vi "Test RT Interpreter API-RT.vi"() -> ()   [LabVIEW 2021]
doc: "RT Interpreter API Tester for Real-Time."
uses:
  Host/Host Interpreter/Host Initialization--cluster.ctl
  Libraries/UDP Comms/UDP Message--cluster.ctl
  <vilib>/Utility/error.llb/DialogType.ctl
  RT Interpreter.lvlib
  Libraries/Common RT/Common RT.lvlib
  Libraries/UDP Comms/UDP Comms.lvlib
panel:
  in  "UDP Message":T1
  in  "Send Message to Host":bool
  in  "Host Initialization--cluster":T2
  out "List of IP:Port:Master/Slave":string[](array[string])
  in  "Exit":bool
  in  "Refresh Modules":bool
  in  "Stop Module Instance":bool
  in  "Run New Module Instance":bool
  out "error out":errorcluster
  out "last error":errorcluster
  out "Active Modules":string[](array[string])
  in  "Select Module":i32(ring)=-1 caption="Select Module\nTo send Request to" items=["All"=-1, "1"=1]
  out "Status":string
  # "This VI tests the API for the Module."
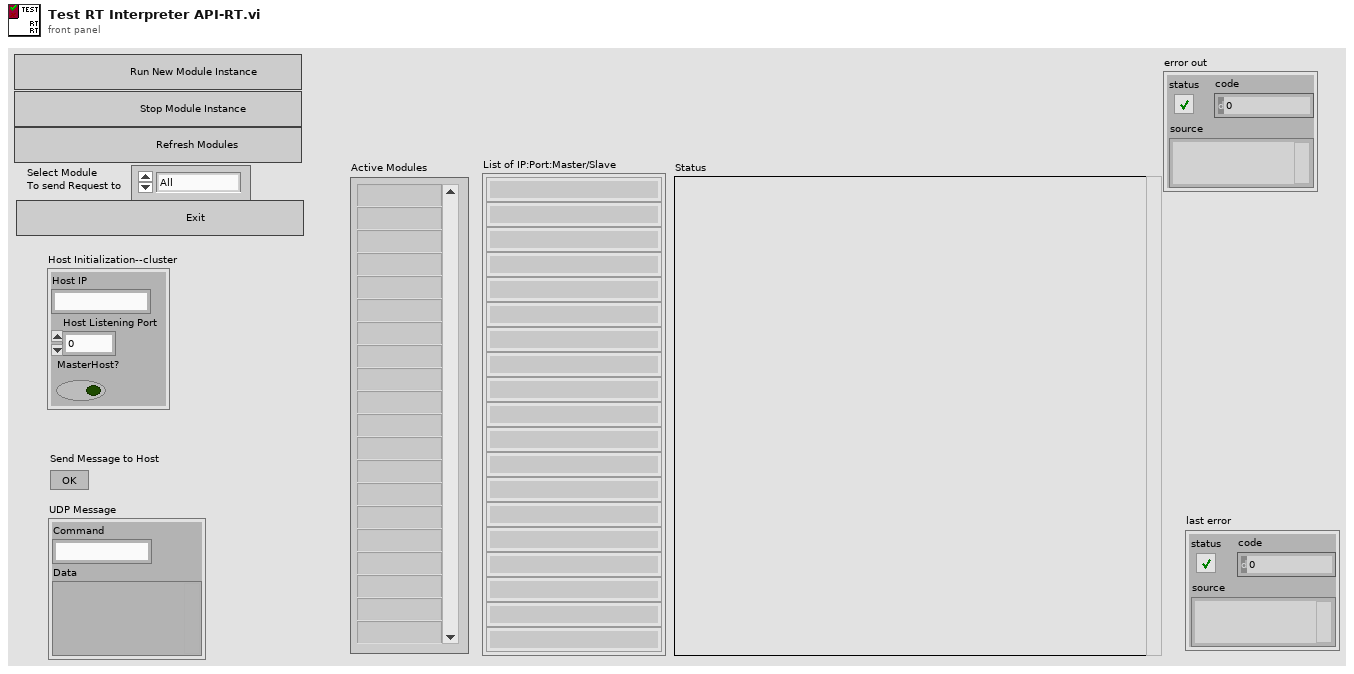
[diagram p1: front panel]
types:
  T1 = typedef "UDP Comms.lvlib/UDP Message--cluster.ctl" = cluster{"Command":string, "Data":variant}
  T2 = typedef "UDP Comms.lvlib/Host Initialization--cluster.ctl" = cluster{"Host IP":string, "Host Listening Port":u16, "MasterHost?":bool}
  T3 = typedef "RT Interpreter.lvlib/Broadcast Events--cluster.ctl" = cluster{"Module Did Init":refnum<user-event>, "Status Updated":refnum<user-event>, "Error Reported":refnum<user-event>, "Module Did Stop":refnum<user-event>, "Update Module Execution Status":refnum<user-event>}
  T4 = typedef "DialogType.ctl" = u16
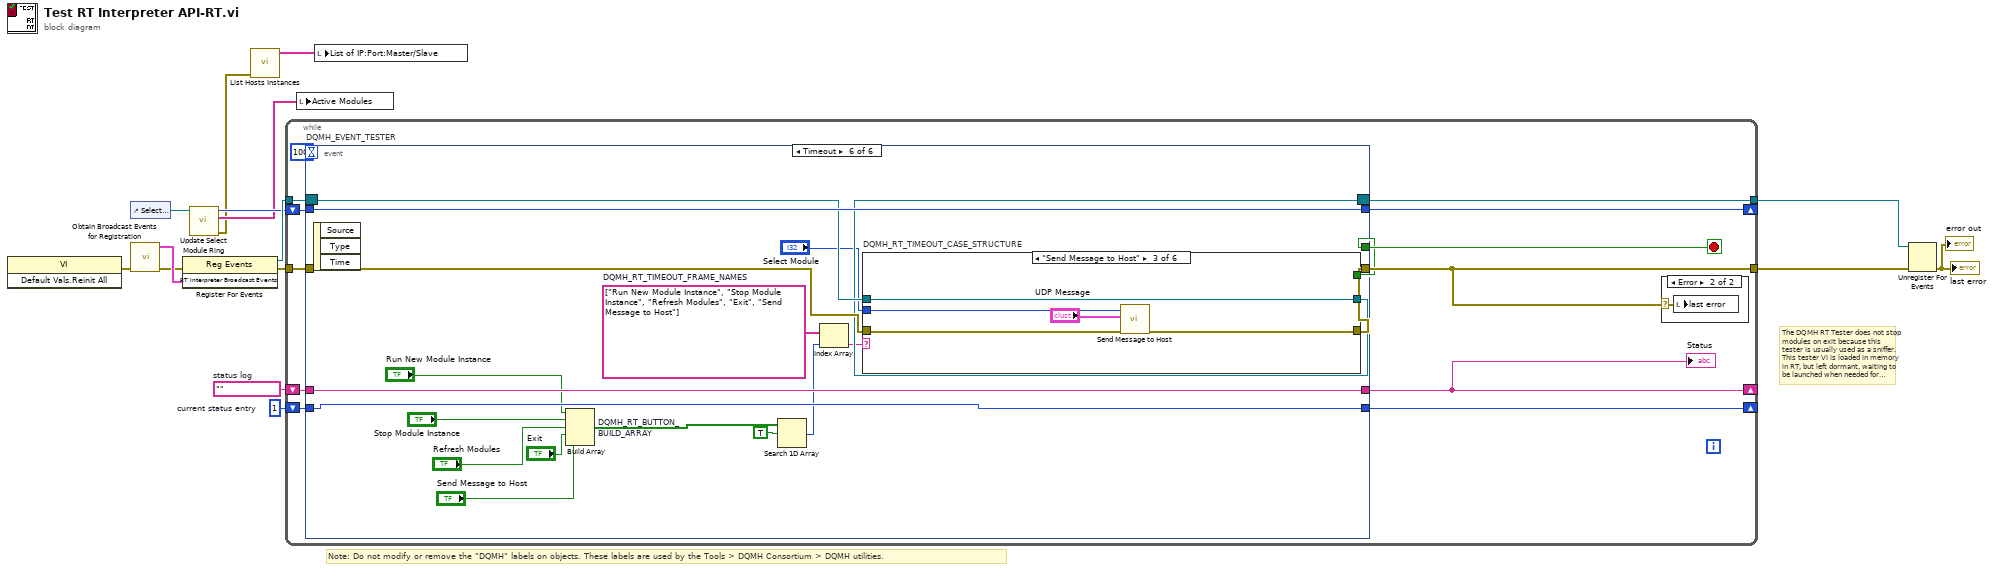
[diagram p0: block diagram]
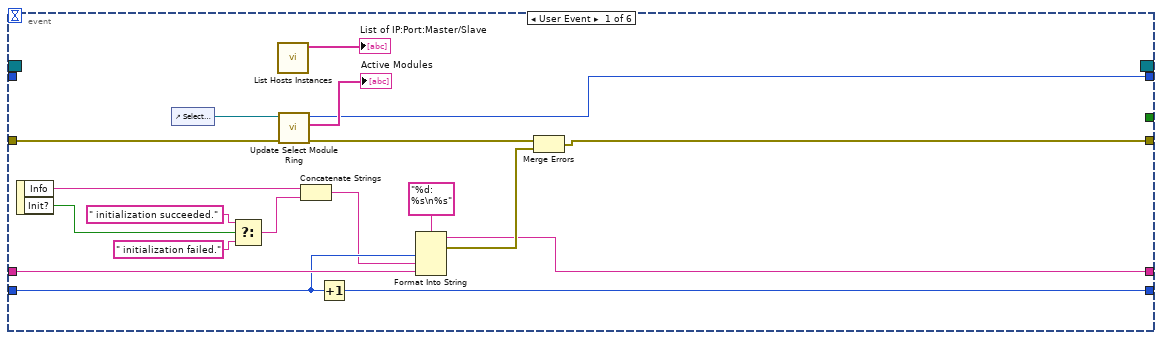
[diagram p3: hidden frame]
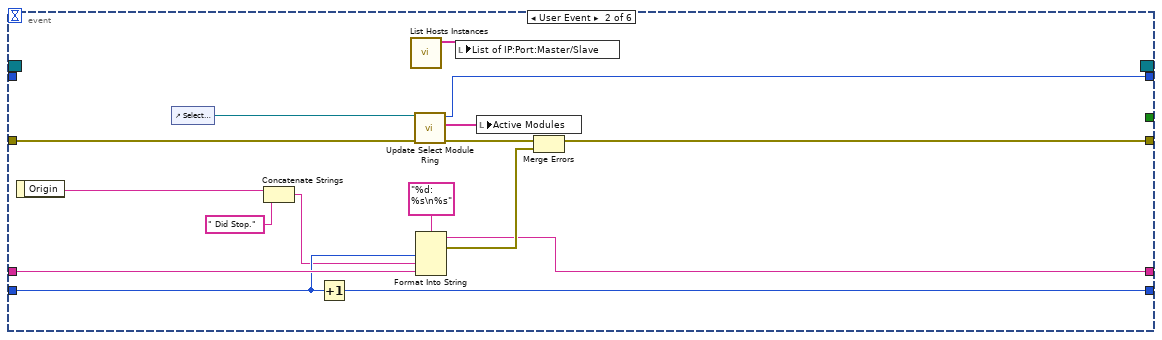
[diagram p4: hidden frame]
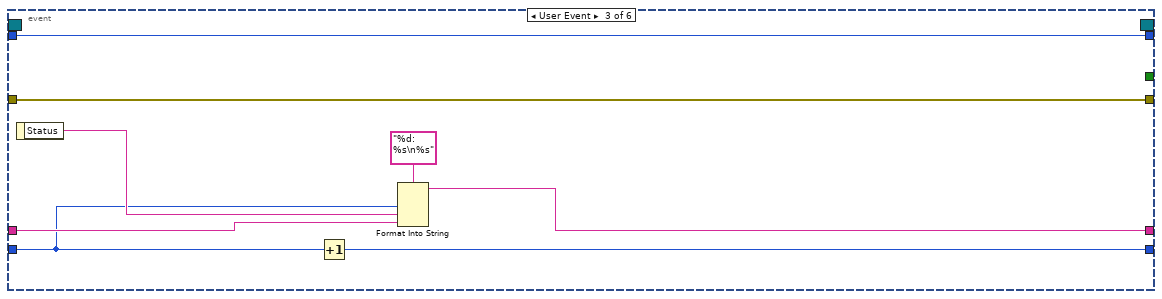
[diagram p5: hidden frame]
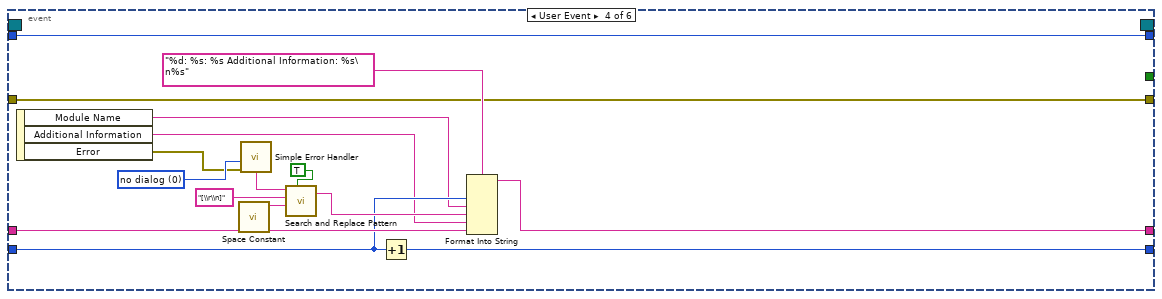
[diagram p6: hidden frame]
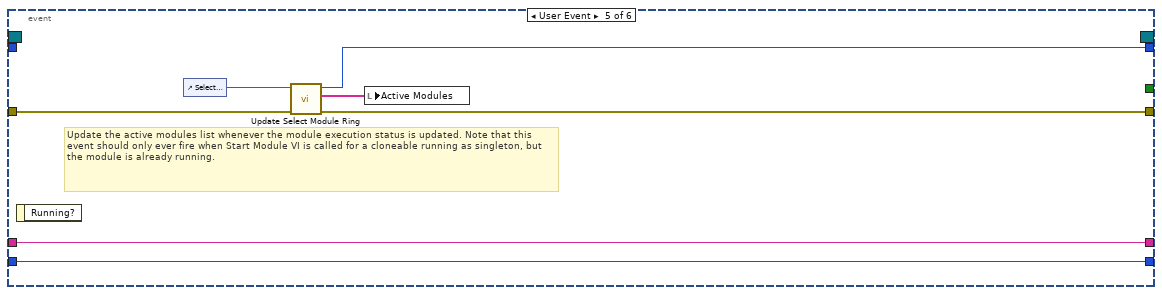
[diagram p7: hidden frame]
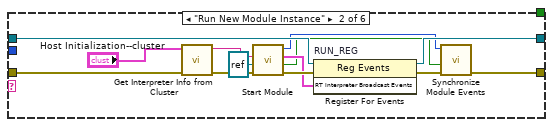
[diagram p9: hidden frame]
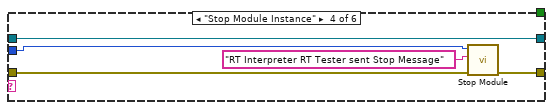
[diagram p10: hidden frame]
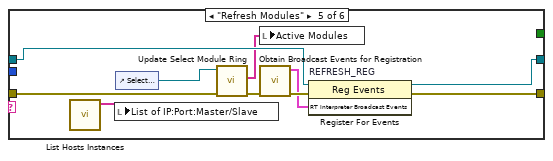
[diagram p11: hidden frame]
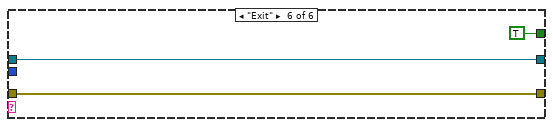
[diagram p12: hidden frame]
diagram:
  w13 = 1  # current status entry
  w14 = ""  # status log
  # "The DQMH RT Tester does not stop modules on exit because this tester is usually used as a sniffer. This tester VI is loaded in memory in RT, but left dormant, waiting to be launched when needed for troubleshooting."
  # "Note: Do not modify or remove the \"DQMH\" labels on objects. These labels are used by the Tools > DQMH Consortium > DQMH utilities."
  n1 = invoke class="VI" method="Default Vals.Reinit All"() -> (error out=w9:errorcluster)  [unwired: 3 in, 2 out]
  n2 = control-ref of="Select Module"() -> (w5:refnum<vi>)
  n3 = call "Obtain Broadcast Events for Registration.vi"("error in"=w9) -> ("error out"=w8:errorcluster, "RT Interpreter Broadcast Events"=w12:T3)  [unwired: 8 in, 1 out]
  n4 = register-events(error in=w8, w12) -> (reference out=w15:refnum<event-registration>, error out=w11:errorcluster)  [unwired: 1 in]
  n5 = call "Update Select Module Ring.vi"("Select Module Ring Ref"=w5) -> ("error out"=w1:errorcluster, "Active Modules (Array)"=w3:string[], "New Module Ring Value"=w4:i32)  [unwired: 8 in]
  n6 = call "List Hosts Instances.vi"("error in"=w1) -> ("List of IP:Port:Master/Slave"=w2:string[])  [unwired: 9 in, 1 out]
  n7 = while {
    tunnel: w15 -> [w27]
    tunnel: [w18] -> w7
    tunnel: w11 -> [w26]
    shift-right: [w22] -> _
    shift-left: w14 -> [w24]
    shift-right: [w23] -> _
    shift-left: w13 -> [w25]
    shift-right: [w20] -> _
    shift-left: w4 -> [w21]
    tunnel: [w19] -> w10
    stop <- w17 stop-if-true
    n8 = event "DQMH_EVENT_TESTER" shown="[5] Timeout" {
      selector: w27 -> [_ _ _ _ _ w108]
      dyn-events: [_ _ _ _ _ w107] -> w19
      timeout: 100 -> [_ _ _ _ _ _]
      tunnel: [_ _ _ _ _ w101] -> w17
      tunnel: [w37 w55 w71 w75 w90 w109] -> w18
      tunnel: w26 -> [w39 w57 w71 w75 w91 w113]
      tunnel: w25 -> [w44 w60 w64 w78 w93 w111]
      tunnel: w24 -> [w45 w61 w67 w79 w94 w112]
      tunnel: [w42 w58 w68 w77 w94 w112] -> w22
      tunnel: [w43 w59 w70 w76 w93 w111] -> w23
      tunnel: w21 -> [_ _ w65 w87 _ w110]
      tunnel: [w34 w52 w65 w87 w89 w110] -> w20
      event User Event {
        n9 = event-data() -> ("Info"=w41:string, "Init?"=w31:bool)  [unwired: 1 in]
        n10 = control-ref of="Select Module"() -> (w36:refnum<vi>)
        n11 = Select(t=" initialization succeeded.", s=w31, f=" initialization failed.") -> (s? t:f=w30:string)
        n12 = call "List Hosts Instances.vi"() -> ("List of IP:Port:Master/Slave"=→"List of IP:Port:Master/Slave":string[])  [unwired: 10 in, 1 out]
        n13 = call "Update Select Module Ring.vi"("error in"=w39, "Select Module Ring Ref"=w36) -> ("error out"=w38:errorcluster, "Active Modules (Array)"=→"Active Modules":string[], "New Module Ring Value"=w34:i32)  [unwired: 7 in]
        n14 = Concatenate Strings(w41, w30) -> (w40:string)
        n15 = Increment(x=w44) -> (x+1=w43:i32)
        n16 = Format Into String(format string="%d: %s\n%s", w44, w40, w45) -> (resulting string=w42:string, error out=w47:errorcluster)  [unwired: 2 in]
        n17 = Merge Errors(w38, w47) -> (w37:errorcluster)
      }
      event User Event {
        n18 = event-data() -> ("Origin"=w50:string)  [unwired: 1 in]
        n19 = control-ref of="Select Module"() -> (w54:refnum<vi>)
        n20 = Concatenate Strings(w50, " Did Stop.") -> (w49:string)
        n21 = Increment(x=w60) -> (x+1=w59:i32)
        n22 = call "List Hosts Instances.vi"() -> ("List of IP:Port:Master/Slave"=w48:string[])  [unwired: 10 in, 1 out]
        n23 = call "Update Select Module Ring.vi"("error in"=w57, "Select Module Ring Ref"=w54) -> ("error out"=w56:errorcluster, "Active Modules (Array)"=w53:string[], "New Module Ring Value"=w52:i32)  [unwired: 7 in]
        n24 = Format Into String(format string="%d: %s\n%s", w60, w49, w61) -> (resulting string=w58:string, error out=w63:errorcluster)  [unwired: 2 in]
        n25 = local write "List of IP:Port:Master/Slave"(w48) -> ()
        n26 = local write "Active Modules"(w53) -> ()
        n27 = Merge Errors(w56, w63) -> (w55:errorcluster)
      }
      event User Event {
        n28 = event-data() -> ("Status"=w66:string)  [unwired: 1 in]
        n29 = Increment(x=w64) -> (x+1=w70:i32)
        n30 = Format Into String(format string="%d: %s\n%s", w64, w66, w67) -> (resulting string=w68:string)  [unwired: 2 in, 1 out]
      }
      event User Event {
        w80 = T4 0 items=["no dialog", "OK message", "continue or stop message", "OK message + warnings", "continue/stop + warnings"] ("type of dialog (OK msg:1)")
        n31 = event-data() -> ("Module Name"=w74:string, "Additional Information"=w73:string, "Error"=w72:errorcluster)  [unwired: 1 in]
        n32 = call <vilib>:"Space Constant.vi"() -> ("String"=w84:string)
        n33 = call <vilib>:"Simple Error Handler.vi"("type of dialog (OK msg:1)"=w80, "error in (no error)"=w72) -> ("message"=w81:string)  [unwired: 3 in, 4 out]
        n34 = call <vilib>:"Search and Replace Pattern.vi"("string"=w81, "regular expression (\"\")"="[\\r\\n]" ("regular expression (\"\")"), "replace string (\"\")"=w84, "replace all? (F)"=TRUE ("replace all CR/LF with spaces")) -> ("result string"=w82:string)  [unwired: 1 in, 1 out]
        n35 = Increment(x=w78) -> (x+1=w76:i32)
        n36 = Format Into String(format string="%d: %s: %s Additional Information: %s\n%s", w78, w74, w82, w73, w79) -> (resulting string=w77:string)  [unwired: 2 in, 1 out]
      }
      event User Event {
        # "Update the active modules list whenever the module execution status is updated. Note that this event should only ever fire when Start Module VI is called for a cloneable running as singleton, but the module is already running."
        n37 = event-data() -> ()  [unwired: 1 in, 1 out]
        n38 = control-ref of="Select Module"() -> (w92:refnum<vi>)
        n39 = call "Update Select Module Ring.vi"("error in"=w91, "Select Module Ring Ref"=w92) -> ("error out"=w90:errorcluster, "Active Modules (Array)"=w88:string[], "New Module Ring Value"=w89:i32)  [unwired: 7 in]
        n40 = local write "Active Modules"(w88) -> ()
      }
      event Timeout {
        w99 = string[] ["Run New Module Instance", "Stop Module Instance", "Refresh Modules", "Exit", "Send Message to Host"]  # DQMH_RT_TIMEOUT_FRAME_NAMES
        n41 = event-data() -> ()  [unwired: 1 in, 3 out]
        n42 = Build Array "DQMH_RT_BUTTON_BUILD_ARRAY"("Run New Module Instance", "Stop Module Instance", "Refresh Modules", "Exit", "Send Message to Host") -> (w96:bool[])
        n43 = Search 1D Array(1D array=w96, element=TRUE) -> (index of element=w98:i32)  [unwired: 1 in]
        n44 = Index Array(array=w99, index=w98) -> (element=w100:string)
        n45 = case "DQMH_RT_TIMEOUT_CASE_STRUCTURE" shown="\"Send Message to Host\"" w100 {
          tunnel: w113 -> [w115 w120 w132 w137 w145 w151]
          tunnel: "Select Module" -> [_ _ w130 w134 _ _]
          tunnel: [w115 w123 w131 w136 w148 w151] -> w109
          tunnel: w108 -> [w114 w127 w133 w138 w147 w150]
          tunnel: [w114 w126 w133 w138 w146 w150] -> w107
          tunnel: [_ _ _ _ _ TRUE] -> w101
          frame "", Default {
          }
          frame "Run New Module Instance" {
            n46 = call "Get Interpreter Info from Cluster.vi"("error in"=w120, "Host Initialization--cluster"="Host Initialization--cluster") -> ("error out"=w119:errorcluster, "IP:Port:Master/Slave"=w118:string)  [unwired: 8 in]
            n47 = call "Start Module.vi"("error in"=w119, "Target UDP connection ref"=refnum<k16> refnum, "IP:Port:Master/Slave"=w118) -> ("error out"=w125:errorcluster, "Wait for Event Sync?"=w122:bool, "RT Interpreter Broadcast Events"=w124:T3, "Module ID"=w121:i32)  [unwired: 4 in, 1 out]
            n48 = register-events "RUN_REG"(reference=w127, error in=w125, w124) -> (reference out=w126:refnum<event-registration>, error out=w128:errorcluster)
            n49 = call "Synchronize Module Events.vi"("error in"=w128, "Wait for Event Sync?"=w122, "Module ID in"=w121) -> ("error out"=w123:errorcluster)  [unwired: 7 in, 1 out]
          }
          frame "Send Message to Host" {
            n50 = call "Send Message to Host.vi"("error in"=w132, "UDP Message"="UDP Message", "Module ID"=w130) -> ("error out"=w131:errorcluster)  [unwired: 8 in]
          }
          frame "Stop Module Instance" {
            n51 = call "Stop Module.vi"("error in"=w137, "Origin"="RT Interpreter RT Tester sent Stop Message", "Module ID"=w134) -> ("error out"=w136:errorcluster)  [unwired: 8 in]
          }
          frame "Refresh Modules" {
            n52 = call "List Hosts Instances.vi"() -> ("List of IP:Port:Master/Slave"=w139:string[])  [unwired: 10 in, 1 out]
            n53 = local write "List of IP:Port:Master/Slave"(w139) -> ()
            n54 = control-ref of="Select Module"() -> (w140:refnum<vi>)
            n55 = call "Update Select Module Ring.vi"("error in"=w145, "Select Module Ring Ref"=w140) -> ("error out"=w142:errorcluster, "Active Modules (Array)"=w141:string[])  [unwired: 7 in, 1 out]
            n56 = local write "Active Modules"(w141) -> ()
            n57 = call "Obtain Broadcast Events for Registration.vi"("error in"=w142) -> ("error out"=w144:errorcluster, "RT Interpreter Broadcast Events"=w143:T3)  [unwired: 8 in, 1 out]
            n58 = register-events "REFRESH_REG"(reference=w147, error in=w144, w143) -> (reference out=w146:refnum<event-registration>, error out=w148:errorcluster)
          }
          frame "Exit" {
          }
        }
      }
    }
    "Status" <- w22
    n59 = case shown="Error" w18 {
      selector: w18 -> [_ w28]
      frame No Error {
      }
      frame Error {
        n60 = local write "last error"(w28) -> ()
      }
    }
  }
  n61 = local write "Active Modules"(w3) -> ()
  n62 = local write "List of IP:Port:Master/Slave"(w2) -> ()
  n63 = Unregister For Events(event registration refnum=w10, error in=w7) -> (error out=→"last error" →"error out":errorcluster)
